vi "ROSToQueue.vi"(3 "Wait?":bool, 4 "ROS":T1={"topic port"=0, "Node"="", "topic"="", "type"="", "node port"=0, "error "={"status"=FALSE, "code"=0, "source"=""}, "Direction"=enum."Node", "APIs"=[], "Update (ms)"=1, "write queue"=1}, 5 "Name":enum16{"topic", "node"}(ring)) -> (0 "Available?":bool, 1 "queue":refnum<queue>)   [LabVIEW 2012]
uses:
  SubVIs/_ROSDirection.ctl
  SubVIs/_ROSControl.ctl
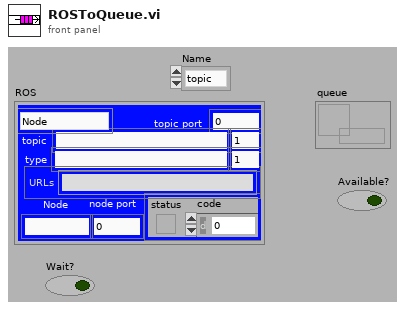
[diagram p1: front panel]
types:
  T1 = typedef "_ROSControl.ctl" = cluster{"topic port":u16, "Node":string, "topic":string, "type":string, "node port":u32, "error ":errorcluster, "Direction":T2, "APIs":string[], "Update (ms)":u16, "write queue":u16}
  T2 = typedef "_ROSDirection.ctl" = enum16{"Node", "Publisher", "Subscriber", "Service Client"}
  T3 = typedef "ServoInfo.ctl" = cluster{"vi name":string, "VI Refnum":refnum<vi>, "queue":refnum<queue>, "ROS":T1, "notifier":refnum<notifier>}
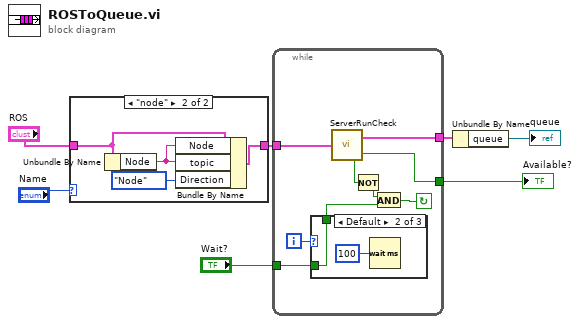
[diagram p0: block diagram]
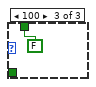
[diagram p3: hidden frame]
diagram:
  n1 = case shown="\"node\"" "Name" {
    tunnel: [w8 w11] -> w3
    tunnel: "ROS" -> [w8 w12]
    frame "topic", Default {
    }
    frame "node" {
      n2 = Unbundle By Name(w12) -> ("Node"=w9:string)
      n3 = Bundle By Name(cluster=w12, "Node"=w9, "topic"=w9, "Direction"=_ROSDirection."Node") -> (w11:T1)
    }
  }
  n4 = while {
    tunnel: [w20] -> w7
    tunnel: [w18] -> w5
    tunnel: w3 -> [w19]
    tunnel: "Wait?" -> [w13]
    i -> [w15]
    stop <- w16 continue-if-true
    n5 = case shown="Default" w15 {
      tunnel: [w21 w22 FALSE ("Wait?")] -> w14
      tunnel: w13 -> [w21 w22 _]
      frame 0 {
      }
      frame Default {
        n6 = Wait (ms)(milliseconds to wait=u32 100) -> ()  [unwired: 1 out]
      }
      frame 100 {
      }
    }
    n7 = call "ServerRunCheck.vi"("ROS in"=w19) -> ("Running?"=w18:bool, "ServerFound"=w20:T3)
    n8 = Not(x=w18) -> (.not. x?=w17:bool)
    n9 = And(x=w17, y=w14) -> (x .and. y?=w16:bool)
  }
  "Available?" <- w5
  n10 = Unbundle By Name(w7) -> ("queue"=→"queue":refnum<queue>)
